vi "Calibration Operation.vi"(0 "VISA resource name":refnum<visa-resource-name>, 1 "Year (2006)":i32=2006, 2 "Month (1)":i32=1, 3 "Day (1)":i32=1, 5 "Type Of Reference (0: Oscillator)":i32(ring) items=["Oscillator", "Voltage"], 7 "Type Of Action (0: Load Factory Calibration )":i32(ring) items=["Load Factory Calibration", "Load User Calibration", "Store User Calibration", "Initialize Calibration"], 11 "error in (no error)":errorcluster) -> (4 "VISA resource name out":refnum<visa-resource-name>, 15 "error out":errorcluster)   [LabVIEW 2019, in "Pendulum CNT90.lvlib"]
doc: "Recalls the calibration factors last stored by the user or factory, or ends the calibration process and stores the calibration factors, or initializes the calibration process."
uses:
  Pendulum CNT90.lvlib
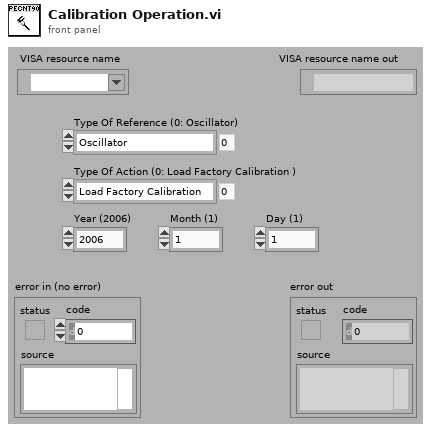
[diagram p1: front panel]
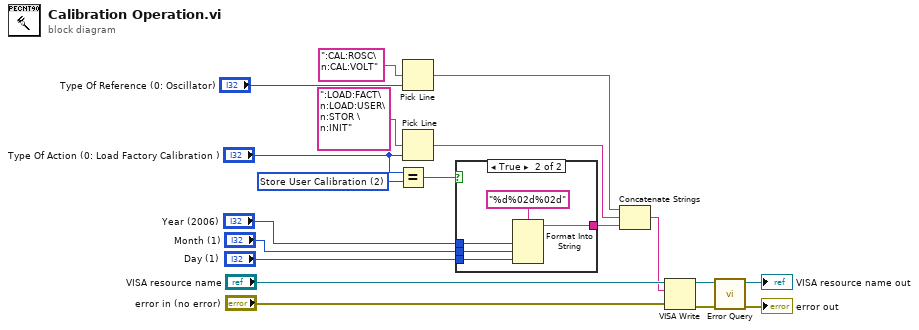
[diagram p0: block diagram]
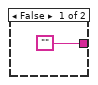
[diagram p2: hidden frame]
diagram:
  w10 = 2 items=["Load Factory Calibration", "Load User Calibration", "Store User Calibration", "Initialize Calibration"] ("Type of Action (0: ) 2")
  n1 = Equal?(x="Type Of Action (0: Load Factory Calibration )", y=w10) -> (x = y?=w8:bool)
  n2 = Pick Line(multi-line string=":CAL:ROSC\n:CAL:VOLT", line index="Type Of Reference (0: Oscillator)") -> (output string=w4:string)  [unwired: 1 in]
  n3 = Pick Line(multi-line string=":LOAD:FACT\n:LOAD:USER\n:STOR \n:INIT", line index="Type Of Action (0: Load Factory Calibration )") -> (output string=w3:string)  [unwired: 1 in]
  n4 = case shown="True" w8 {
    tunnel: "Year (2006)" -> [_ w24]
    tunnel: "Month (1)" -> [_ w23]
    tunnel: "Day (1)" -> [_ w22]
    tunnel: ["" w21] -> w2
    frame False {
    }
    frame True {
      n5 = Format Into String(format string="%d%02d%02d", w24, w23, w22) -> (resulting string=w21:string)  [unwired: 2 in, 1 out]
    }
  }
  n6 = Concatenate Strings(w4, w3, w2) -> (w1:string)
  n7 = VISA Write(VISA resource name="VISA resource name", write buffer=w1, error in (no error)="error in (no error)") -> (VISA resource name out=w17:refnum<visa-resource-name>, error out=w14:errorcluster)  [unwired: 1 out]
  n8 = call "Error Query.vi"("error in (no error)"=w14, "VISA resource name"=w17) -> ("error out"=→"error out":errorcluster, "VISA resource name out"=→"VISA resource name out":refnum<visa-resource-name>)  [unwired: 6 in, 2 out]
